vi "FileExplorerQueueDriver.vi"(0 "Queue Name":string, 5 "Enqueue Element":T1, 7 "Enqueue N Element":T1[](array[typedef]), 11 "error in (no error)":errorcluster, 13 "Enum":T2) -> (4 "Dequeue Element":T1, 15 "error out":errorcluster)   [LabVIEW 2023]
doc: "Used as queue driver to perform various queue operations like create queue, enqueue, dequeue, flush and close queue."
uses:
  TypeDefs/FileExplorerQueueOperations.ctl
  TypeDefs/FileExplorerStateDataCluster.ctl
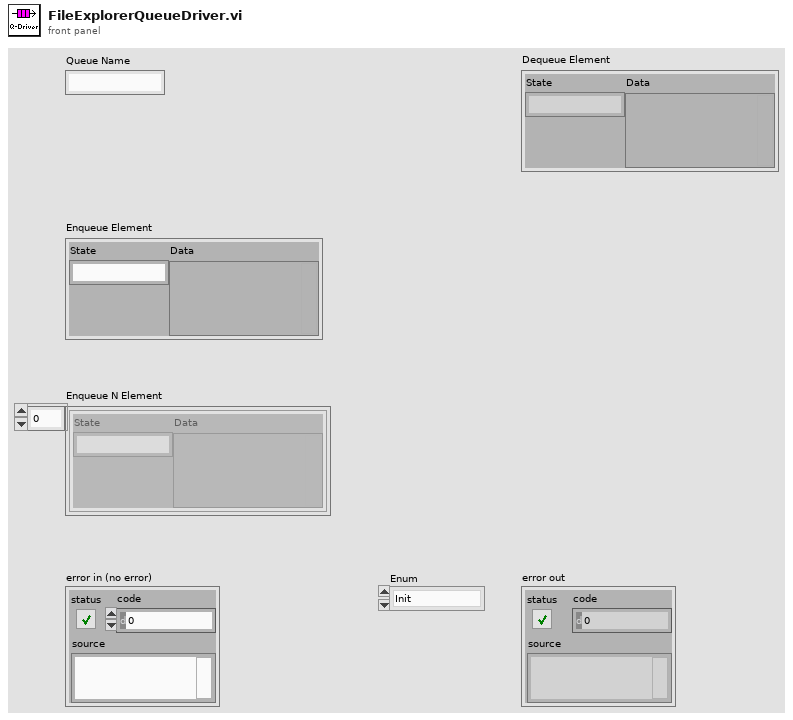
[diagram p1: front panel]
types:
  T1 = typedef "FileExplorerStateDataCluster.ctl" = cluster{"State":string, "Data":variant}
  T2 = typedef "FileExplorerQueueOperations.ctl" = enum16{"Init", "Enqueue", "Dequeue", "Enqueue N", "Flush", "Close", "Enqueue N Stack"}
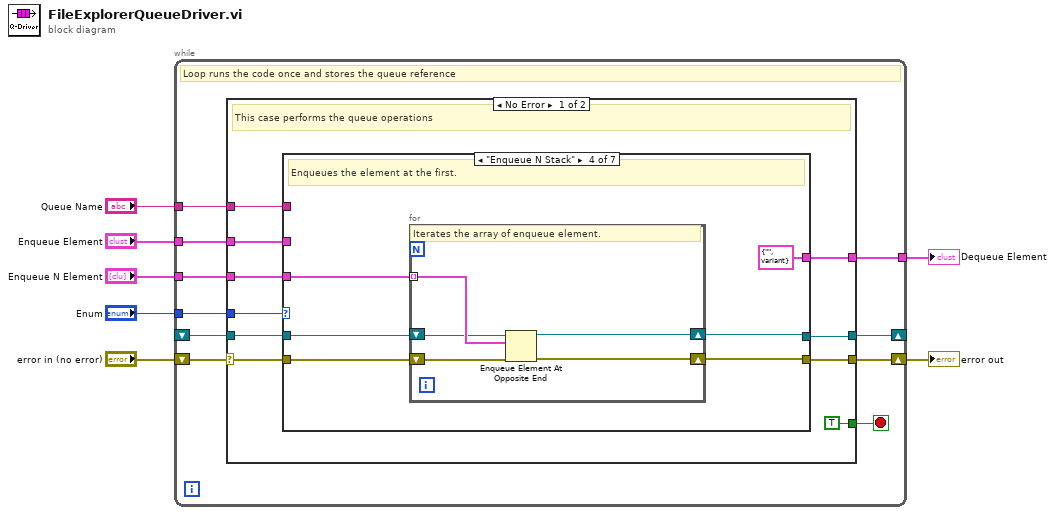
[diagram p0: block diagram]
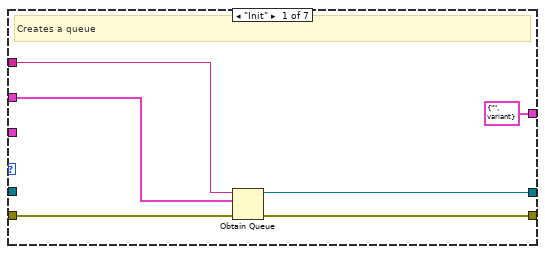
[diagram p2: hidden frame]
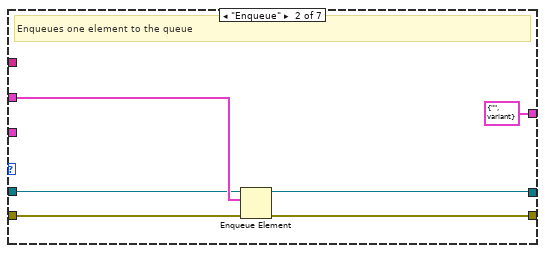
[diagram p3: hidden frame]
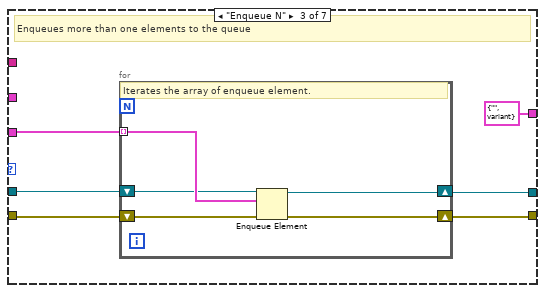
[diagram p4: hidden frame]
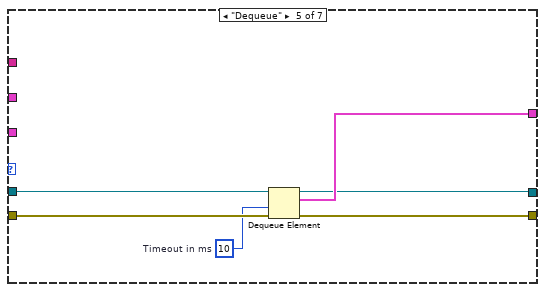
[diagram p5: hidden frame]
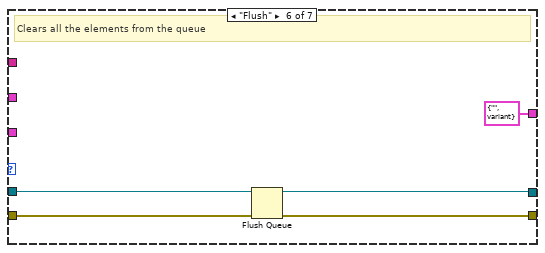
[diagram p6: hidden frame]
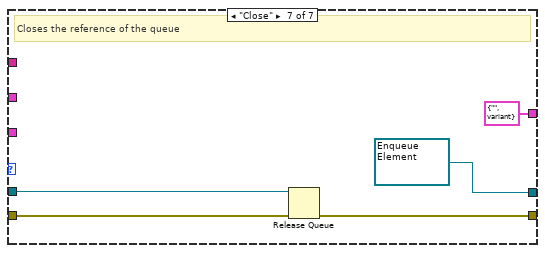
[diagram p7: hidden frame]
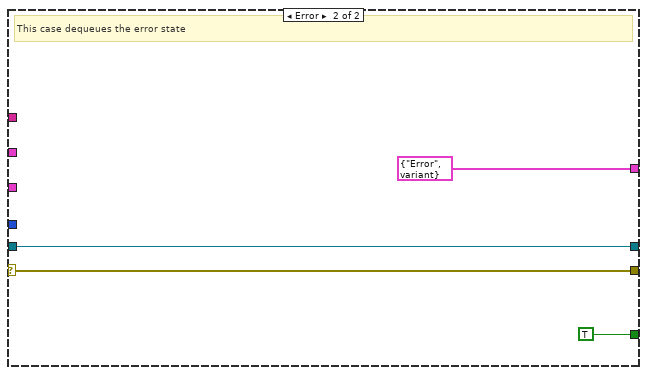
[diagram p8: hidden frame]
diagram:
  n1 = while {
    tunnel: "Queue Name" -> [w15]
    tunnel: "Enum" -> [w14]
    tunnel: "Enqueue N Element" -> [w13]
    tunnel: "Enqueue Element" -> [w12]
    tunnel: [w11] -> w1
    shift-right: [w10] -> _
    shift-left: _ -> [w9]
    shift-right: [w16] -> w6
    shift-left: "error in (no error)" -> [w17]
    stop <- w8 stop-if-true
    # "Loop runs the code once and stores the queue reference"
    n2 = case shown="No Error" w17 {
      selector: w17 -> [w26 w81]
      tunnel: w15 -> [w27 _]
      tunnel: [w25 w81] -> w16
      tunnel: w14 -> [w24 _]
      tunnel: w13 -> [w23 _]
      tunnel: w12 -> [w22 _]
      tunnel: [w21 T1 {"State"="Error", "Data"=variant} ("Enqueue Element")] -> w11
      tunnel: [w20 w79] -> w10
      tunnel: w9 -> [w19 w79]
      tunnel: [TRUE TRUE] -> w8
      frame No Error {
        # "This case performs the queue operations"
        n3 = case shown="\"Enqueue N Stack\"" w24 {
          tunnel: w27 -> [w31 _ _ _ _ _ _]
          tunnel: w26 -> [w33 w39 w44 w56 w67 w72 w77]
          tunnel: [w32 w38 w43 w55 w66 w71 w76] -> w25
          tunnel: w23 -> [_ _ w45 w53 _ _ _]
          tunnel: w22 -> [w30 w37 _ _ _ _ _]
          tunnel: [T1 {"State"="", "Data"=variant} ("Enqueue Element") T1 {"State"="", "Data"=variant} ("Enqueue Element") T1 {"State"="", "Data"=variant} ("Enqueue Element") T1 {"State"="", "Data"=variant} ("Enqueue Element") w65 T1 {"State"="", "Data"=variant} ("Enqueue Element") T1 {"State"="", "Data"=variant} ("Enqueue Element")] -> w21
          tunnel: [w29 w35 w41 w52 w63 w69 refnum<queue> refnum ("queue out")] -> w20
          tunnel: w19 -> [_ w36 w42 w54 w64 w70 w75]
          frame "Init" {
            # "Creates a queue"
            n4 = Obtain Queue(name (unnamed)=w31, element data type=w30, error in (no error)=w33) -> (queue out=w29:refnum<queue>, error out=w32:errorcluster)  [unwired: 2 in, 1 out]
          }
          frame "Enqueue" {
            # "Enqueues one element to the queue"
            n5 = Enqueue Element(queue=w36, element=w37, error in (no error)=w39) -> (queue out=w35:refnum<queue>, error out=w38:errorcluster)  [unwired: 1 in, 1 out]
          }
          frame "Enqueue N" {
            # "Enqueues more than one elements to the queue"
            n6 = for {
              tunnel: w45 -> [w48] mode=indexing
              shift-right: [w47] -> w41
              shift-left: w42 -> [w46]
              shift-right: [w49] -> w43
              shift-left: w44 -> [w50]
              # "Iterates the array of enqueue element."
              n7 = Enqueue Element(queue=w46, element=w48, error in (no error)=w50) -> (queue out=w47:refnum<queue>, error out=w49:errorcluster)  [unwired: 1 in, 1 out]
            }
          }
          frame "Enqueue N Stack" {
            # "Enqueues the element at the first."
            n8 = for {
              shift-right: [w60] -> w55
              shift-left: w56 -> [w61]
              tunnel: w53 -> [w59] mode=indexing
              shift-right: [w57] -> w52
              shift-left: w54 -> [w58]
              # "Iterates the array of enqueue element."
              n9 = Enqueue Element At Opposite End(queue=w58, element=w59, error in (no error)=w61) -> (queue out=w57:refnum<queue>, error out=w60:errorcluster)  [unwired: 1 in, 1 out]
            }
          }
          frame "Dequeue" {
            w62 = 10  # Timeout in ms
            n10 = Dequeue Element(queue=w64, timeout in ms (-1)=w62, error in (no error)=w67) -> (queue out=w63:refnum<queue>, element=w65:T1, error out=w66:errorcluster)  [unwired: 1 out]
          }
          frame "Flush" {
            # "Clears all the elements from the queue"
            n11 = Flush Queue(queue=w70, error in (no error)=w72) -> (queue out=w69:refnum<queue>, error out=w71:errorcluster)  [unwired: 1 out]
          }
          frame "Close" {
            # "Closes the reference of the queue"
            n12 = Release Queue(queue=w75, error in (no error)=w77) -> (error out=w76:errorcluster)  [unwired: 1 in, 2 out]
          }
        }
      }
      frame Error {
        # "This case dequeues the error state"
      }
    }
  }
  "error out" <- w6
  "Dequeue Element" <- w1
